vi "initializeDefaultStyle.vi"(8 "error in (no error)":errorcluster, 11 "Heading 3 in":refnum<class "Heading 3.lvclass">) -> (0 "error out":errorcluster, 3 "Heading 3 out":refnum<class "Heading 3.lvclass">)   [LabVIEW 2017, in "Styles.lvlib" / "Heading 3.lvclass"]
uses:
  Heading 3.lvclass
  C:/Users/Neo/Desktop/Dev_Tools_BR/LabVIEW_NPOI/src/Styles/Style/Style.lvclass
  Heading/Heading.lvclass
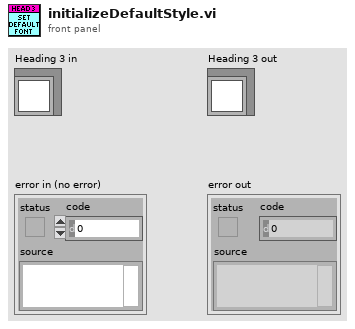
[diagram p1: front panel]
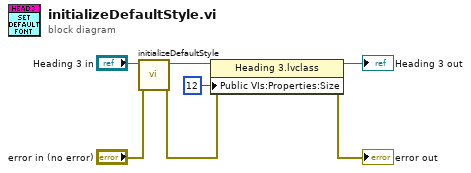
[diagram p0: block diagram]
diagram:
  n1 = call-parent "initializeDefaultStyle.vi"("error in (no error)"="error in (no error)", "Heading in"="Heading 3 in") -> ("error out"=w3:errorcluster, "Heading out"=w7:refnum<class "Heading 3.lvclass">)  [unwired: 8 in]
  n2 = property class="Heading 3.lvclass"(reference=w7, error in=w3, "Public VIs:Properties:Size"=12 ("Style:Size")) -> (reference out=→"Heading 3 out":refnum<class "Heading 3.lvclass">, error out=→"error out":errorcluster)
